vi "VisitLVAnalogWaveformType.vi"(8 "error in (no error)":errorcluster, 10 "LVAnalogWaveformType":refnum<class "LVAnalogWaveformType.lvclass">, 11 "NextGenXMLTypeGenerator in":refnum<class "NextGenXMLTypeGenerator.lvclass">) -> (0 "error out":errorcluster, 3 "NextGenXMLTypeGenerator out":refnum<class "NextGenXMLTypeGenerator.lvclass">)   [LabVIEW 2020, in "Web Service Description.lvlib" / "NextGenXMLTypeGenerator.lvclass"]
uses:
  <vilib>/AppBuilder/Engine/WebServiceDescription/NextGenXMLTypeGenerator/NextGenXMLTypeGenerator.lvclass
  e:/builds/penguin/labview/branches/2020/dev/dist/vi.lib/AppBuilder/Engine/WebServiceDescription/LVDataTypes/LVTypeVisitor/LVTypeVisitor.lvclass
  <vilib>/AppBuilder/Engine/WebServiceDescription/LVDataTypes/LVAnalogWaveformType/LVAnalogWaveformType.lvclass
  <vilib>/AppBuilder/Engine/WebServiceDescription/XMLGen/ValuePair.ctl
  <vilib>/AppBuilder/Engine/WebServiceDescription/NextGenXMLTypeGenerator/NextGenXMLTypeGenerator.lvclass/NextGenXMLTypeGenerator.ctl
  <vilib>/AppBuilder/Engine/WebServiceDescription/GetTypeAttributesVisitor/GetTypeAttributesVisitor.lvclass
  <vilib>/AppBuilder/Engine/WebServiceDescription/LVDataTypes/LVType/LVType.lvclass
  <vilib>/AppBuilder/Engine/WebServiceDescription/XMLGen/XMLGen.lvlib
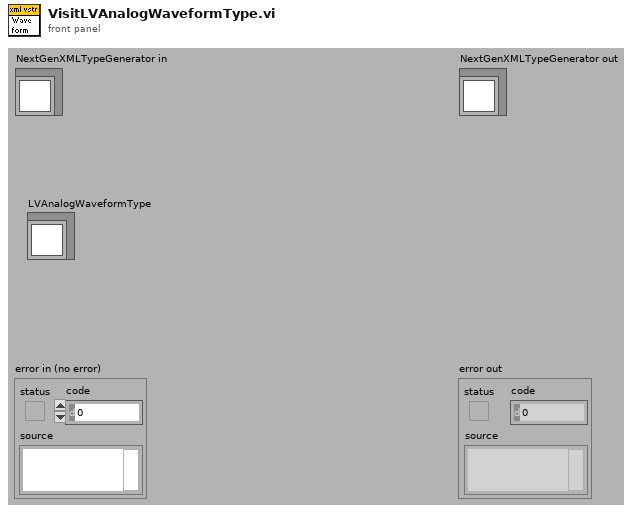
[diagram p1: front panel]
types:
  T1 = typedef "XMLGen.lvlib/ValuePair.ctl" = cluster{"Name":string, "Value":string}
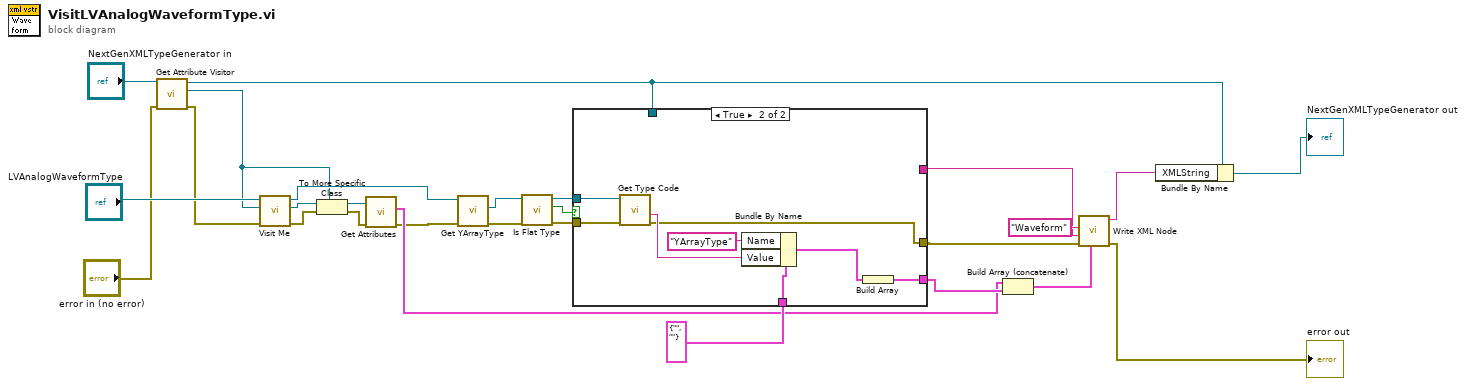
[diagram p0: block diagram]
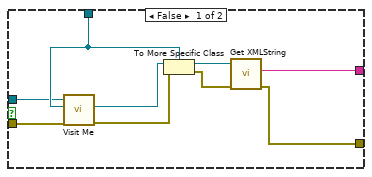
[diagram p2: hidden frame]
diagram:
  n1 = call <vilib>:"Get Attribute Visitor.vi"("error in (no error)"="error in (no error)", "NextGenXMLTypeGenerator in"="NextGenXMLTypeGenerator in") -> ("error out"=w3:errorcluster, "Attribute Visitor"=w2:refnum<class "GetTypeAttributesVisitor.lvclass">, "NextGenXMLTypeGenerator out"=w1:refnum<class "NextGenXMLTypeGenerator.lvclass">)  [unwired: 7 out]
  n2 = call-dynamic "Visit Me.vi"("error in (no error)"=w3, "Visitor In"=w2, "LVAnalogWaveformType in"="LVAnalogWaveformType") -> ("error out"=w12:errorcluster, "Visitor Out"=w13:refnum<class "LVTypeVisitor.lvclass">, "LVAnalogWaveformType out"=w8:refnum<class "LVAnalogWaveformType.lvclass">)  [unwired: 6 out]
  n3 = To More Specific Class(target class=w2, reference=w13, error in=w12) -> (specific class reference=w10:refnum<class "GetTypeAttributesVisitor.lvclass">, error out=w11:errorcluster)
  n4 = call <vilib>:"Get Attributes.vi"("error in (no error)"=w11, "GetTypeAttributesVisitor.lvclass in"=w10) -> ("error out"=w6:errorcluster, "Attributes"=w7:T1[])  [unwired: 8 out]
  n5 = call <vilib>:"Get YArrayType.vi"("error in (no error)"=w6, "LVAnalogWaveformType.lvclass in"=w8) -> ("error out"=w18:errorcluster, "YArrayType"=w17:refnum<class "LVType.lvclass">)  [unwired: 8 out]
  n6 = call-dynamic "Is Flat Type.vi"("error in (no error)"=w18, "LVType in"=w17) -> ("error out"=w22:errorcluster, "Flat Type?"=w21:bool, "LVType out"=w23:refnum<class "LVType.lvclass">)  [unwired: 7 out]
  n7 = case shown="True" w21 {
    tunnel: [w36 w37] -> w19
    tunnel: [w35 _] -> w20
    tunnel: w1 -> [w30 _]
    tunnel: w22 -> [w29 w44]
    tunnel: w23 -> [w28 w43]
    tunnel: T1 {"Name"="", "Value"=""} ("Attribute") -> [_ w41]
    tunnel: [_ w38] -> w15
    frame False {
      n8 = call-dynamic "Visit Me.vi"("error in (no error)"=w29, "Visitor In"=w30, "LVType in"=w28) -> ("error out"=w32:errorcluster, "Visitor Out"=w31:refnum<class "LVTypeVisitor.lvclass">)  [unwired: 7 out]
      n9 = To More Specific Class(target class=w30, reference=w31, error in=w32) -> (specific class reference=w33:refnum<class "NextGenXMLTypeGenerator.lvclass">, error out=w34:errorcluster)
      n10 = call <vilib>:"Get XMLString.vi"("error in (no error)"=w34, "NextGenXMLTypeGenerator.lvclass in"=w33) -> ("error out"=w36:errorcluster, "XMLString"=w35:string)  [unwired: 8 out]
    }
    frame True {
      n11 = call <vilib>:"Get Type Code.vi"("error in (no error)"=w44, "LVType.lvclass in"=w43) -> ("error out"=w37:errorcluster, "TypeCodeString"=w40:string)  [unwired: 8 out]
      n12 = Bundle By Name(cluster=w41, "Name"="YArrayType", "Value"=w40) -> (w39:T1)
      n13 = Build Array(w39) -> (w38:T1[])
    }
  }
  n14 = Build Array (concatenate)(w7, w15) -> (w14:T1[])
  n15 = call <vilib>:"Write XML Node.vi"("attributes"=w14, "error in (no error)"=w19, "body"=w20, "node"="Waveform") -> ("error out"=→"error out":errorcluster, "resulting string"=w25:string)  [unwired: 1 in, 5 out]
  n16 = Bundle By Name(cluster=w1, "XMLString"=w25) -> (→"NextGenXMLTypeGenerator out":refnum<class "NextGenXMLTypeGenerator.lvclass">)
